vi "PH_4_Pos_Selector.set GUI Elements for the first time.vi"(0 "VI in":refnum<vi>, 5 "error in (no error)":errorcluster) -> (14 "VI out":refnum<vi>, 19 "error out":errorcluster)   [LabVIEW 2014, in "PH_4_Pos_Selector.lvlib"]
uses:
  PH_4_Pos_Selector.lvlib
  PH_Basics/PH_Common/PH_Common.lvlib
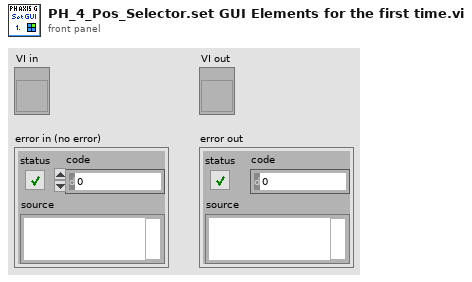
[diagram p1: front panel]
types:
  T1 = typedef "PH_4_Pos_Selector.lvlib/PH_4_Pos_Selector.i attribute.ctl" = cluster{"GUI Refs":cluster{"Position I":refnum<vi>, "Position II":refnum<vi>, "Position III":refnum<vi>, "Position IV":refnum<vi>, "rel. Mode?":refnum<vi>, "Define Selector":refnum<vi>}, "Current Position":T2, "Service ID Position":i32, "Position Array":T3[], "Description Array":string[], "relative Mode":bool, "Wanted Define Selector Position":string}
  T2 = typedef "PH_4_Pos_Selector.lvlib/PH_4_Pos_Selector.Position Selector.ctl" = u16
  T3 = typedef "PH_4_Pos_Selector.lvlib/PH_4_Pos_Selector.Position.ctl" = cluster{"Axis 1":dbl, "Axis 2":dbl}
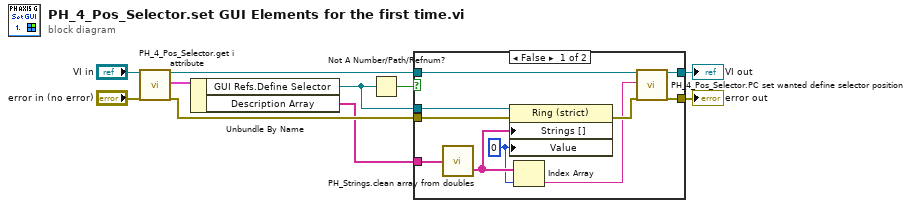
[diagram p0: block diagram]
diagram:
  n1 = call "PH_4_Pos_Selector.get i attribute.vi"("i ref in"="VI in", "error in (no error)"="error in (no error)") -> ("i ref out"=w10:refnum<vi>, "i attribute"=w6:T1, "error out"=w8:errorcluster)  [unwired: 15 in]
  n2 = Unbundle By Name(w6) -> ("GUI Refs.Define Selector"=w2:refnum<vi>, "Description Array"=w5:string[])
  n3 = Not A Number/Path/Refnum?(number/path/refnum=w2) -> (NaN/Path/Refnum?=w1:bool)
  n4 = case shown="False" w1 {
    tunnel: w10 -> [w13 w22]
    tunnel: w8 -> [w20 w21]
    tunnel: w2 -> [w19 _]
    tunnel: w5 -> [w18 _]
    tunnel: [w15 w22] -> w4
    tunnel: [w14 w21] -> w3
    frame False {
      w16 = 0 ("Value")
      n5 = call "PH_Strings.clean array from doubles.vi"("Array Input"=w18) -> ("Cleaned Array Output"=w17:string[])  [unwired: 1 out]
      n6 = property class="Ring (strict)"(reference=w19, error in=w20, "Strings []"=w17, "Value"=w16) -> (error out=w12:errorcluster)  [unwired: 1 out]
      n7 = Index Array(array=w17, index=w16) -> (element=w11:string)
      n8 = call "PH_4_Pos_Selector.PC set wanted define selector position.vi"("VI in"=w13, "Wanted Define Selector Position"=w11, "error in (no error)"=w12) -> ("VI out"=w15:refnum<vi>, "error out"=w14:errorcluster)  [unwired: 15 in]
    }
    frame True {
    }
  }
  "VI out" <- w4
  "error out" <- w3
